vi "UpdateStock.vi"(1 "id_produit":string, 2 "quantite":dbl) -> (0 "Result Set":string[][](table))   [LabVIEW 2024]
uses:
  <vilib>/drjdpowell/SQLite Library/SQL Connection/Open (string).vi
  <vilib>/drjdpowell/SQLite Library/SQL Connection/Execute SQL.vi
  <vilib>/drjdpowell/SQLite Library/SQL Connection/Connection.lvclass
  <vilib>/drjdpowell/SQLite Library/SQLite.lvlib
panel:
  # "Update Stock"
  # "Etat de Stock"
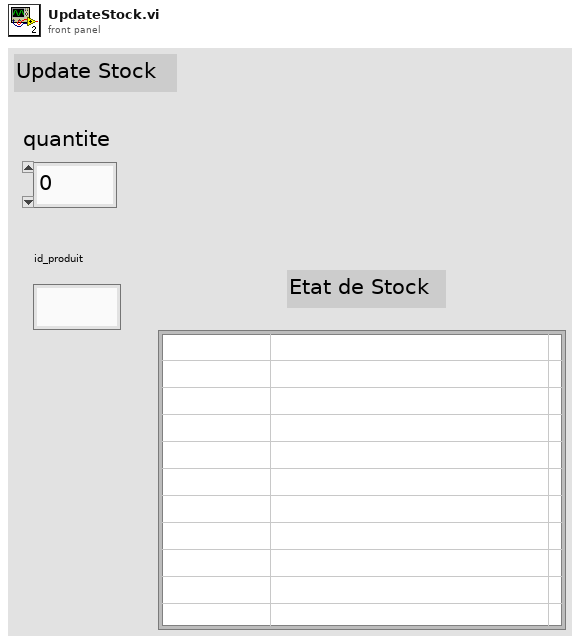
[diagram p1: front panel]
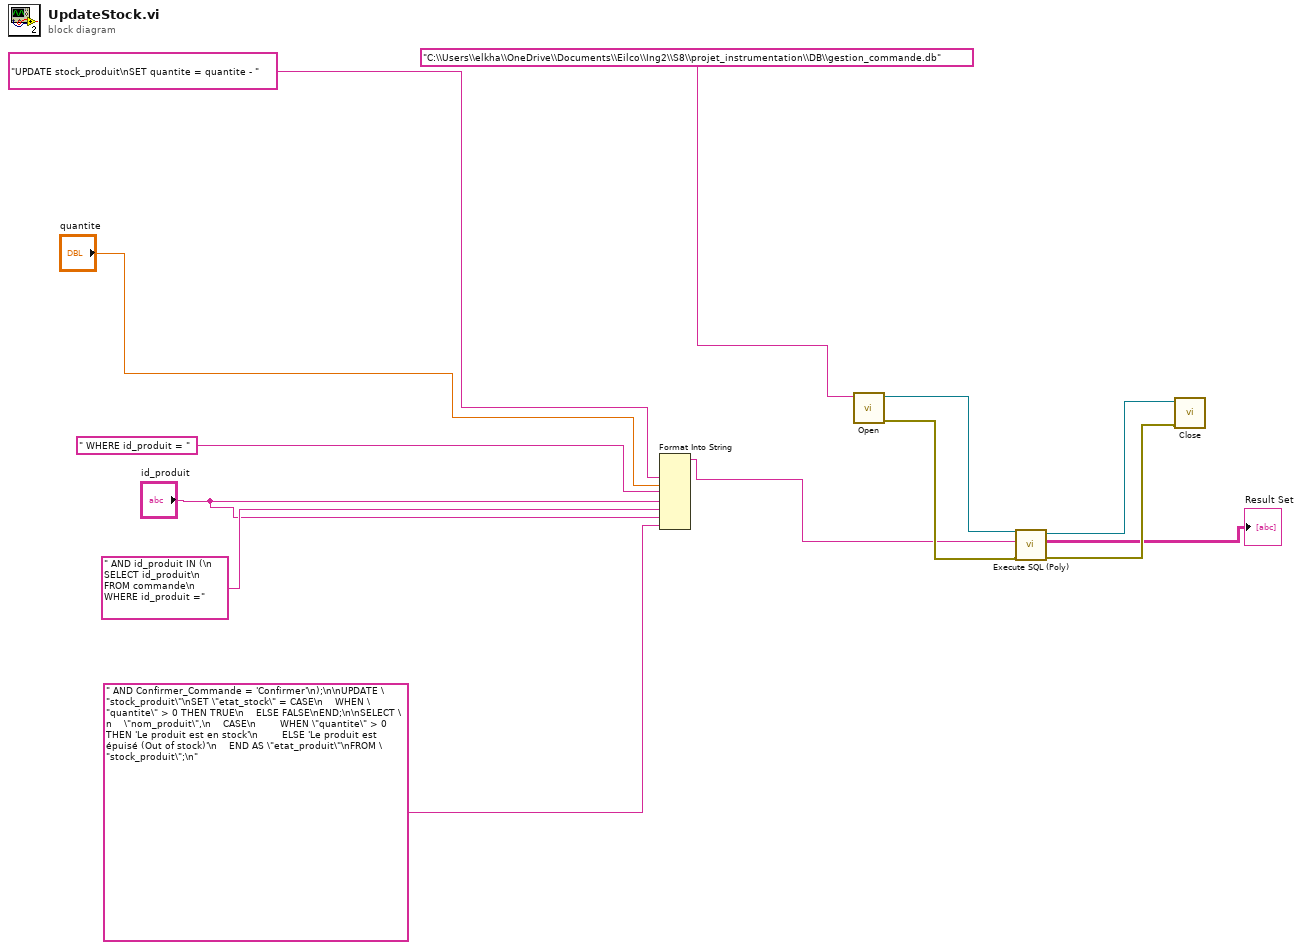
[diagram p0: block diagram]
diagram:
  n1 = Format Into String("UPDATE stock_produit\nSET quantite = quantite - ", "quantite", " WHERE id_produit = ", "id_produit", " AND id_produit IN (\n    SELECT id_produit\n    FROM commande\n    WHERE id_produit =", "id_produit", " AND Confirmer_Commande = 'Confirmer'\n);\n\nUPDATE \"stock_produit\"\nSET \"etat_stock\" = CASE\n    WHEN \"quantite\" > 0 THEN TRUE\n    ELSE FALSE\nEND;\n\nSELECT \n    \"nom_produit\",\n    CASE\n        WHEN \"quantite\" > 0 THEN 'Le produit est en stock'\n        ELSE 'Le produit est épuisé (Out of stock)'\n    END AS \"etat_produit\"\nFROM \"stock_produit\";\n") -> (resulting string=w8:string)  [unwired: 3 in, 1 out]
  n2 = call-poly <vilib>:"Open.vi"("db file"="C:\\Users\\elkha\\OneDrive\\Documents\\Eilco\\Ing2\\S8\\projet_instrumentation\\DB\\gestion_commande.db") -> ("error out"=w10:errorcluster, "SQLite Connection"=w13:refnum<class "Connection.lvclass">)  [unwired: 9 in]
  n3 = call-poly <vilib>:"Execute SQL (Poly).vi"("error in (no error)"=w10, "SQL"=w8, "SQLite Connection in"=w13) -> ("error out"=w11:errorcluster, "Result Set"=→"Result Set":string[][], "SQLite Connection"=w12:refnum<class "Connection.lvclass">)  [unwired: 5 in, 1 out]
  n4 = call-dynamic "Close.vi"("error in (no error)"=w11, "SQLite Connection in"=w12) -> ()  [unwired: 9 in, 1 out]
